vi "console_panel.vi"() -> ()   [LabVIEW 2012]
doc: "This VI is to serve as a simplified version of the utility_panel.vi, demonstrating primarily the ability to communicate with the connected device via the ASCII commandset.\n\nProduced By:\n\nChristopher Lemieux\nKod Integrations, LLC\n4835 Marianne Drive\nMount Airy, MD 21771\nhttp://www.kodintegrations.com\nemail: clemieux@kodintegrations.com\nphone: (240) 687-1288"
uses:
  support/controls/utility_actions.ctl
  main_functions/commands.ctl
  support/controls/errors_actions.ctl
panel:
  in  "help":bool
  out "response":string
  in  "terminate":bool
  in  "raw_cmd":string
  in  "write_cmd":bool
  out "error out":errorcluster
  in  "error in (no error)":errorcluster
  # "COMMAND:"
  # "RESPONSE:"
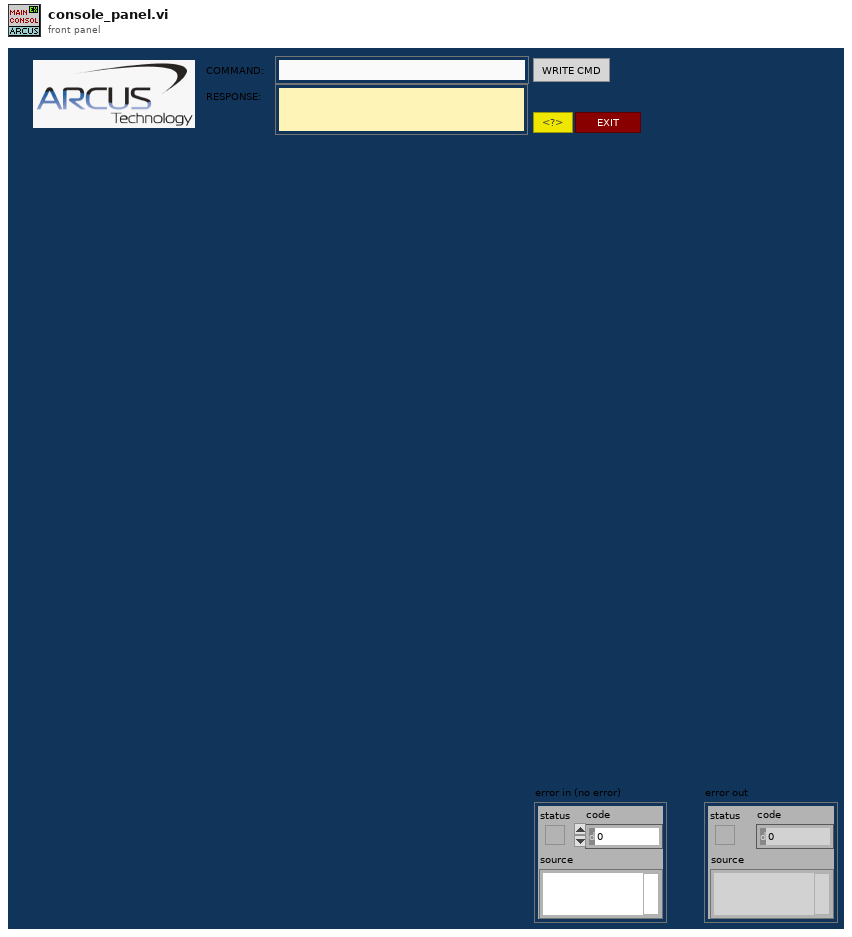
[diagram p1: front panel]
types:
  T1 = typedef "utility_actions.ctl" = enum16{"about", "clearError", "closeRef", "demo", "getAcceleration", "getActualCurrentVal", "getDeviceId", "getDeviceList", "getDigInputs", "getDigOutputs", "getDriverPowerStatus", "getFirmwareVer", "getHighSpeed", "getIdleCurrent", "getLowSpeed", "getMode", "getPolarity", "getPosition", "getProductId", "getRunCurrent", "getStatus", "homeMotorNeg", "homeMotorPos", "initialize", "jogConstNeg", "jogConstPos", "moveToPos", "openRef", "pause", "powerOFF", "powerON", "processEvents", "rawCmd", "setAcceleration", "setDeviceId", "setDigOutput", "setHighSpeed", "setLowSpeed", "setPolarity", "setPosition", "setRunCurrent", "setIdleCurrent", "setMode", "setTimeOuts", "stopImmediately", "stopSlowly", "storeToFlashMem", "updatePanelItems", "validateDemoPos", "validatePos", "waitUntilDone", "zeroPosition"}
  T2 = typedef "errors_actions.ctl" = enum16{"clearBuff", "closeRef", "noDeviceInfo", "noDevices", "openRef", "sendReceive", "setTimeouts", "unknown"}
  T3 = typedef "commands.ctl" = enum16{"clear error", "constant jog(-)", "constant jog(+)", "get acceleration", "get actual current", "get device id", "get digital input status", "get digial inputs status", "get dig output status", "get digital outputs status", "get firmware ver", "get high speed", "get idle current", "get low speed", "get micro step", "get motor status", "get move mode", "get polarity", "get position", "get product id", "get power status", "get run current", "get status", "home(-)", "home(+)", "move to position", "power down", "power up", "set acceleration", "set device id", "set digital output", "set digital outputs", "set high speed", "set idle current", "set low speed", "set move mode absolute", "set move mode increment", "set polarity", "set position", "set run current", "stop immediate", "stop slow", "store to memory"}
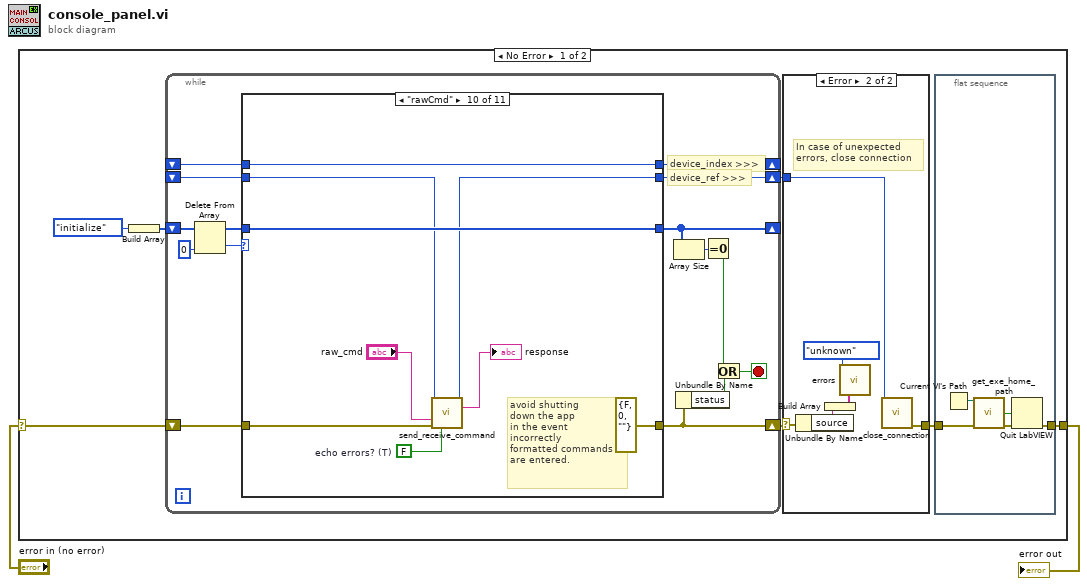
[diagram p0: block diagram]
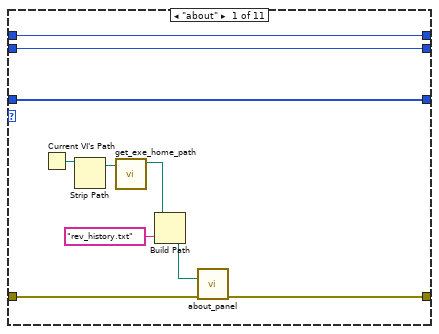
[diagram p3: hidden frame]
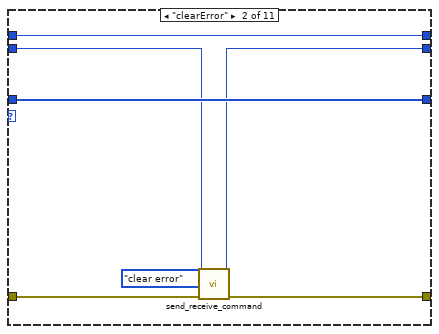
[diagram p4: hidden frame]
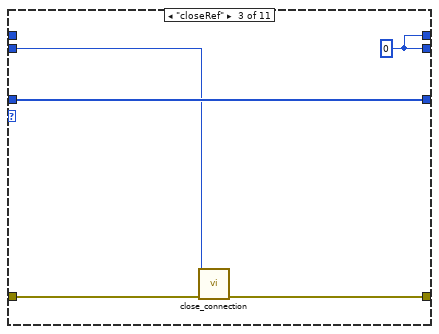
[diagram p5: hidden frame]
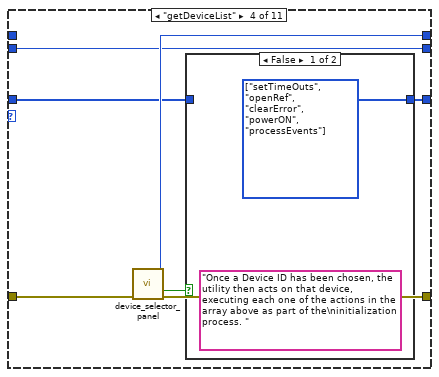
[diagram p6: hidden frame]
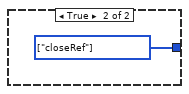
[diagram p7: hidden frame]
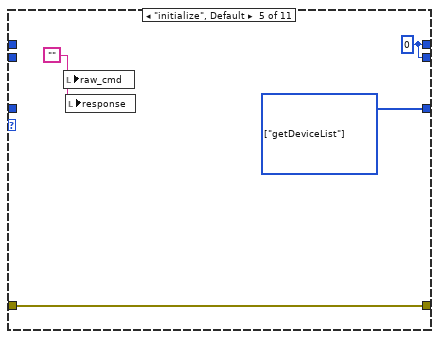
[diagram p8: hidden frame]
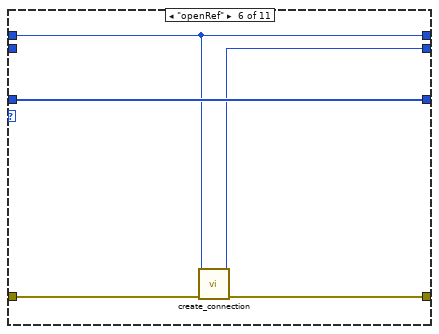
[diagram p9: hidden frame]
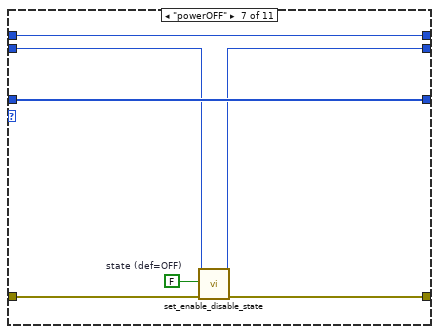
[diagram p10: hidden frame]
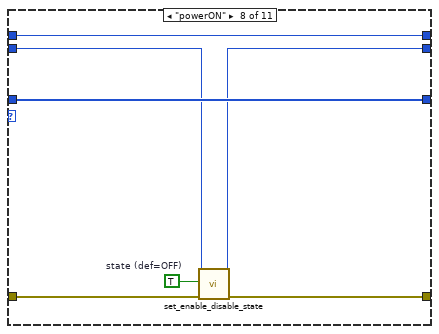
[diagram p11: hidden frame]
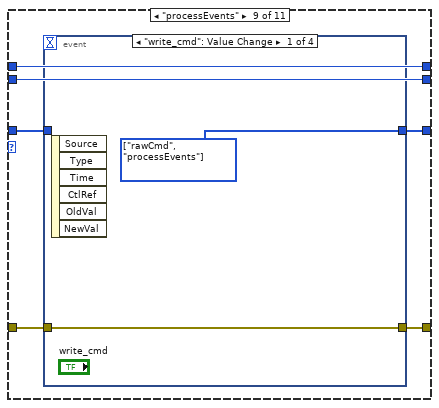
[diagram p12: hidden frame]
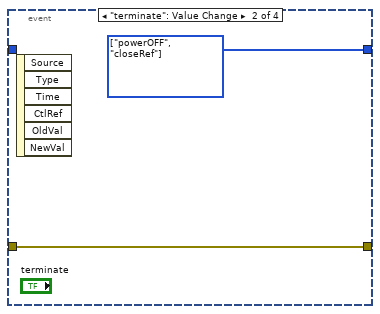
[diagram p13: hidden frame]
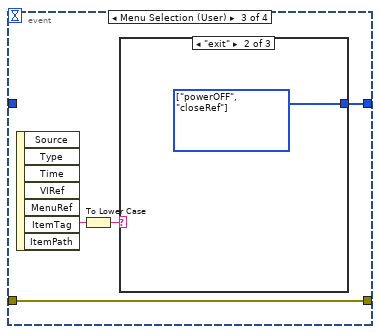
[diagram p14: hidden frame]
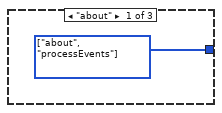
[diagram p15: hidden frame]
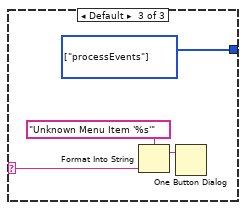
[diagram p16: hidden frame]
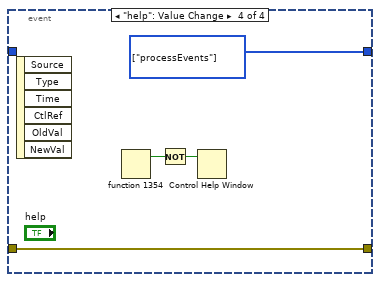
[diagram p17: hidden frame]
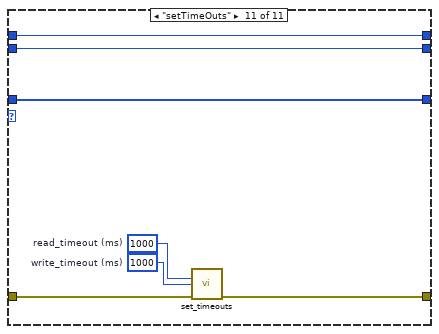
[diagram p18: hidden frame]
diagram:
  n1 = case shown="No Error" "error in (no error)" {
    selector: "error in (no error)" -> [w5 w129]
    tunnel: [w3 w129] -> w1
    frame No Error {
      n2 = Build Array(utility_actions."initialize" ("Enum")) -> (w8:T1[])
      n3 = while {
        shift-right: [w29] -> _
        shift-left: w8 -> [w34]
        shift-right: [w24] -> w7
        shift-left: w5 -> [w30]
        shift-right: [w23] -> w6
        shift-left: _ -> [w22]
        shift-right: [w21] -> _
        shift-left: _ -> [w20]
        stop <- w25 stop-if-true
        # "device_index >>>"
        # "device_ref >>>"
        n4 = Delete From Array(array=w34, index=0) -> (deleted portion=w32:T1, array with subset deleted=w31:T1[])  [unwired: 1 in]
        n5 = case shown="\"rawCmd\"" w32 {
          tunnel: w31 -> [w44 w51 w56 w58 _ w74 w81 w88 w91 w120 w122]
          tunnel: [w44 w51 w56 w57 w68 w74 w81 w88 w92 w120 w122] -> w29
          tunnel: w30 -> [w41 w49 w55 w63 w69 w73 w78 w86 w94 w121 w126]
          tunnel: [w40 w48 w54 w62 w69 w72 w77 w85 w93 errorcluster {"status"=FALSE, "code"=0, "source"=""} w125] -> w24
          tunnel: [w42 w46 w52 w60 w67 w71 w75 w82 w89 w115 w127] -> w23
          tunnel: w22 -> [w42 w47 w53 w60 _ _ w76 w83 w89 w116 w127]
          tunnel: [w43 w50 w52 w61 w67 w70 w80 w87 w90 w117 w128] -> w21
          tunnel: w20 -> [w43 w50 _ _ _ w70 w80 w87 w90 w117 w128]
          frame "about" {
            n6 = Current VI's Path() -> (path=w37:path)
            n7 = Strip Path(path=w37) -> (stripped path=w36:path)  [unwired: 1 out]
            n8 = call "get_exe_home_path.vi"("home_path"=w36) -> ("actual_home_path"=w35:path)  [unwired: 6 in, 1 out]
            n9 = Build Path(base path=w35, name or relative path="rev_history.txt") -> (appended path=w38:path)
            n10 = call "about_panel.vi"("rev_history_filepath"=w38, "error in (no error)"=w41) -> ("error out"=w40:errorcluster)  [unwired: 13 in]
          }
          frame "clearError" {
            n11 = call "send_receive_command.vi"("reference (in)"=w47, "command"=commands."clear error" ("commands"), "error in (no error)"=w49) -> ("reference (dup)"=w46:i32, "error out"=w48:errorcluster)  [unwired: 8 in, 3 out]
          }
          frame "closeRef" {
            w52 = 0 ("reference (out)")
            n12 = call "close_connection.vi"("reference"=w53, "error in (no error)"=w55) -> ("error out"=w54:errorcluster)  [unwired: 13 in]
          }
          frame "getDeviceList" {
            n13 = call "device_selector_panel.vi"("error in (no error)"=w63) -> ("index"=w61:i32, "cancel?"=w59:bool, "error out"=w62:errorcluster)  [unwired: 10 in, 2 out]
            n14 = case shown="False" w59 {
              tunnel: w58 -> [_ _]
              tunnel: [w64 w65] -> w57
              frame False {
                w64 = T1[] [enum."setTimeOuts", enum."openRef", enum."clearError", enum."powerON", enum."processEvents"] items=["about", "clearError", "closeRef", "demo", "getAcceleration", "getActualCurrentVal", "getDeviceId", "getDeviceList", "getDigInputs", "getDigOutputs", "getDriverPowerStatus", "getFirmwareVer", "getHighSpeed", "getIdleCurrent", "getLowSpeed", "getMode", "getPolarity", "getPosition", "getProductId", "getRunCurrent", "getStatus", "homeMotorNeg", "homeMotorPos", "initialize", "jogConstNeg", "jogConstPos", "moveToPos", "openRef", "pause", "powerOFF", "powerON", "processEvents", "rawCmd", "setAcceleration", "setDeviceId", "setDigOutput", "setHighSpeed", "setLowSpeed", "setPolarity", "setPosition", "setRunCurrent", "setIdleCurrent", "setMode", "setTimeOuts", "stopImmediately", "stopSlowly", "storeToFlashMem", "updatePanelItems", "validateDemoPos", "validatePos", "waitUntilDone", "zeroPosition"] ("actions")
                (unwired) "Once a Device ID has been chosen, the utility then acts on that device, executing each one of the actions in the array above as part of the\ninitialization process. "
              }
              frame True {
                w65 = T1[] [enum."closeRef"] items=["about", "clearError", "closeRef", "demo", "getAcceleration", "getActualCurrentVal", "getDeviceId", "getDeviceList", "getDigInputs", "getDigOutputs", "getDriverPowerStatus", "getFirmwareVer", "getHighSpeed", "getIdleCurrent", "getLowSpeed", "getMode", "getPolarity", "getPosition", "getProductId", "getRunCurrent", "getStatus", "homeMotorNeg", "homeMotorPos", "initialize", "jogConstNeg", "jogConstPos", "moveToPos", "openRef", "pause", "powerOFF", "powerON", "processEvents", "rawCmd", "setAcceleration", "setDeviceId", "setDigOutput", "setHighSpeed", "setLowSpeed", "setPolarity", "setPosition", "setRunCurrent", "setIdleCurrent", "setMode", "setTimeOuts", "stopImmediately", "stopSlowly", "storeToFlashMem", "updatePanelItems", "validateDemoPos", "validatePos", "waitUntilDone", "zeroPosition"] ("actions")
              }
            }
          }
          frame "initialize", Default {
            w68 = T1[] [enum."getDeviceList"] items=["about", "clearError", "closeRef", "demo", "getAcceleration", "getActualCurrentVal", "getDeviceId", "getDeviceList", "getDigInputs", "getDigOutputs", "getDriverPowerStatus", "getFirmwareVer", "getHighSpeed", "getIdleCurrent", "getLowSpeed", "getMode", "getPolarity", "getPosition", "getProductId", "getRunCurrent", "getStatus", "homeMotorNeg", "homeMotorPos", "initialize", "jogConstNeg", "jogConstPos", "moveToPos", "openRef", "pause", "powerOFF", "powerON", "processEvents", "rawCmd", "setAcceleration", "setDeviceId", "setDigOutput", "setHighSpeed", "setLowSpeed", "setPolarity", "setPosition", "setRunCurrent", "setIdleCurrent", "setMode", "setTimeOuts", "stopImmediately", "stopSlowly", "storeToFlashMem", "updatePanelItems", "validateDemoPos", "validatePos", "waitUntilDone", "zeroPosition"] ("actions")
            w67 = 0 ("index")
            w66 = ""
            n15 = local write "raw_cmd"(w66) -> ()
            n16 = local write "response"(w66) -> ()
          }
          frame "openRef" {
            n17 = call "create_connection.vi"("device_index (def=0)"=w70, "error in (no error)"=w73) -> ("reference"=w71:i32, "error out"=w72:errorcluster)  [unwired: 12 in]
          }
          frame "powerOFF" {
            w79 = FALSE  # state (def=OFF)
            n18 = call "set_enable_disable_state.vi"("reference (in)"=w76, "state (def=OFF)"=w79, "error in (no error)"=w78) -> ("reference (dup)"=w75:i32, "error out"=w77:errorcluster)  [unwired: 14 in, 1 out]
          }
          frame "powerON" {
            w84 = TRUE  # state (def=OFF)
            n19 = call "set_enable_disable_state.vi"("reference (in)"=w83, "state (def=OFF)"=w84, "error in (no error)"=w86) -> ("reference (dup)"=w82:i32, "error out"=w85:errorcluster)  [unwired: 14 in, 1 out]
          }
          frame "processEvents" {
            n20 = event shown="[0] \"write_cmd\": Value Change" {
              selector: _ -> [_ _ _ _]
              dyn-events: _ -> [_ _ _ _]
              timeout: _ -> [_ _ _ _]
              tunnel: [w96 w98 w99 w112] -> w93
              tunnel: w94 -> [w96 w98 w99 w112]
              tunnel: [w95 w97 w100 w111] -> w92
              tunnel: w91 -> [_ _ _ _]
              event "write_cmd": Value Change {
                w95 = T1[] [enum."rawCmd", enum."processEvents"] items=["about", "clearError", "closeRef", "demo", "getAcceleration", "getActualCurrentVal", "getDeviceId", "getDeviceList", "getDigInputs", "getDigOutputs", "getDriverPowerStatus", "getFirmwareVer", "getHighSpeed", "getIdleCurrent", "getLowSpeed", "getMode", "getPolarity", "getPosition", "getProductId", "getRunCurrent", "getStatus", "homeMotorNeg", "homeMotorPos", "initialize", "jogConstNeg", "jogConstPos", "moveToPos", "openRef", "pause", "powerOFF", "powerON", "processEvents", "rawCmd", "setAcceleration", "setDeviceId", "setDigOutput", "setHighSpeed", "setLowSpeed", "setPolarity", "setPosition", "setRunCurrent", "setIdleCurrent", "setMode", "setTimeOuts", "stopImmediately", "stopSlowly", "storeToFlashMem", "updatePanelItems", "validateDemoPos", "validatePos", "waitUntilDone", "zeroPosition"] ("actions")
                n21 = event-data() -> ()  [unwired: 1 in, 6 out]
              }
              event "terminate": Value Change {
                w97 = T1[] [enum."powerOFF", enum."closeRef"] items=["about", "clearError", "closeRef", "demo", "getAcceleration", "getActualCurrentVal", "getDeviceId", "getDeviceList", "getDigInputs", "getDigOutputs", "getDriverPowerStatus", "getFirmwareVer", "getHighSpeed", "getIdleCurrent", "getLowSpeed", "getMode", "getPolarity", "getPosition", "getProductId", "getRunCurrent", "getStatus", "homeMotorNeg", "homeMotorPos", "initialize", "jogConstNeg", "jogConstPos", "moveToPos", "openRef", "pause", "powerOFF", "powerON", "processEvents", "rawCmd", "setAcceleration", "setDeviceId", "setDigOutput", "setHighSpeed", "setLowSpeed", "setPolarity", "setPosition", "setRunCurrent", "setIdleCurrent", "setMode", "setTimeOuts", "stopImmediately", "stopSlowly", "storeToFlashMem", "updatePanelItems", "validateDemoPos", "validatePos", "waitUntilDone", "zeroPosition"] ("actions")
                n22 = event-data() -> ()  [unwired: 1 in, 6 out]
              }
              event Menu Selection (User) {
                n23 = event-data() -> ("ItemTag"=w102:string)  [unwired: 1 in, 6 out]
                n24 = To Lower Case(string=w102) -> (all lower case string=w101:string)
                n25 = case shown="\"exit\"" w101 {
                  selector: w101 -> [_ _ w105]
                  tunnel: [w103 w104 w108] -> w100
                  frame "about" {
                    w103 = T1[] [enum."about", enum."processEvents"] items=["about", "clearError", "closeRef", "demo", "getAcceleration", "getActualCurrentVal", "getDeviceId", "getDeviceList", "getDigInputs", "getDigOutputs", "getDriverPowerStatus", "getFirmwareVer", "getHighSpeed", "getIdleCurrent", "getLowSpeed", "getMode", "getPolarity", "getPosition", "getProductId", "getRunCurrent", "getStatus", "homeMotorNeg", "homeMotorPos", "initialize", "jogConstNeg", "jogConstPos", "moveToPos", "openRef", "pause", "powerOFF", "powerON", "processEvents", "rawCmd", "setAcceleration", "setDeviceId", "setDigOutput", "setHighSpeed", "setLowSpeed", "setPolarity", "setPosition", "setRunCurrent", "setIdleCurrent", "setMode", "setTimeOuts", "stopImmediately", "stopSlowly", "storeToFlashMem", "updatePanelItems", "validateDemoPos", "validatePos", "waitUntilDone", "zeroPosition"] ("actions")
                  }
                  frame "exit" {
                    w104 = T1[] [enum."powerOFF", enum."closeRef"] items=["about", "clearError", "closeRef", "demo", "getAcceleration", "getActualCurrentVal", "getDeviceId", "getDeviceList", "getDigInputs", "getDigOutputs", "getDriverPowerStatus", "getFirmwareVer", "getHighSpeed", "getIdleCurrent", "getLowSpeed", "getMode", "getPolarity", "getPosition", "getProductId", "getRunCurrent", "getStatus", "homeMotorNeg", "homeMotorPos", "initialize", "jogConstNeg", "jogConstPos", "moveToPos", "openRef", "pause", "powerOFF", "powerON", "processEvents", "rawCmd", "setAcceleration", "setDeviceId", "setDigOutput", "setHighSpeed", "setLowSpeed", "setPolarity", "setPosition", "setRunCurrent", "setIdleCurrent", "setMode", "setTimeOuts", "stopImmediately", "stopSlowly", "storeToFlashMem", "updatePanelItems", "validateDemoPos", "validatePos", "waitUntilDone", "zeroPosition"] ("actions")
                  }
                  frame Default {
                    w108 = T1[] [enum."processEvents"] items=["about", "clearError", "closeRef", "demo", "getAcceleration", "getActualCurrentVal", "getDeviceId", "getDeviceList", "getDigInputs", "getDigOutputs", "getDriverPowerStatus", "getFirmwareVer", "getHighSpeed", "getIdleCurrent", "getLowSpeed", "getMode", "getPolarity", "getPosition", "getProductId", "getRunCurrent", "getStatus", "homeMotorNeg", "homeMotorPos", "initialize", "jogConstNeg", "jogConstPos", "moveToPos", "openRef", "pause", "powerOFF", "powerON", "processEvents", "rawCmd", "setAcceleration", "setDeviceId", "setDigOutput", "setHighSpeed", "setLowSpeed", "setPolarity", "setPosition", "setRunCurrent", "setIdleCurrent", "setMode", "setTimeOuts", "stopImmediately", "stopSlowly", "storeToFlashMem", "updatePanelItems", "validateDemoPos", "validatePos", "waitUntilDone", "zeroPosition"] ("actions")
                    n26 = Format Into String(format string="Unknown Menu Item '%s'" ("message"), w105) -> (resulting string=w106:string)  [unwired: 2 in, 1 out]
                    n27 = One Button Dialog(message=w106) -> ()  [unwired: 1 in, 1 out]
                  }
                }
              }
              event "help": Value Change {
                w111 = T1[] [enum."processEvents"] items=["about", "clearError", "closeRef", "demo", "getAcceleration", "getActualCurrentVal", "getDeviceId", "getDeviceList", "getDigInputs", "getDigOutputs", "getDriverPowerStatus", "getFirmwareVer", "getHighSpeed", "getIdleCurrent", "getLowSpeed", "getMode", "getPolarity", "getPosition", "getProductId", "getRunCurrent", "getStatus", "homeMotorNeg", "homeMotorPos", "initialize", "jogConstNeg", "jogConstPos", "moveToPos", "openRef", "pause", "powerOFF", "powerON", "processEvents", "rawCmd", "setAcceleration", "setDeviceId", "setDigOutput", "setHighSpeed", "setLowSpeed", "setPolarity", "setPosition", "setRunCurrent", "setIdleCurrent", "setMode", "setTimeOuts", "stopImmediately", "stopSlowly", "storeToFlashMem", "updatePanelItems", "validateDemoPos", "validatePos", "waitUntilDone", "zeroPosition"] ("actions")
                n28 = event-data() -> ()  [unwired: 1 in, 6 out]
                n29 = fn#1354() -> (1:w110:bool)  [unwired: 1 out]
                n30 = Not(x=w110) -> (.not. x?=w109:bool)
                n31 = Control Help Window(1:w109) -> ()  [unwired: 1 in]
              }
            }
          }
          frame "rawCmd" {
            w113 = FALSE  # echo errors? (T)
            # "avoid shutting\ndown the app\nin the event\nincorrectly \nformatted commands\nare entered."
            n32 = call "send_receive_command.vi"("reference (in)"=w116, "command (raw)"="raw_cmd", "error in (no error)"=w121, "echo errors? (T)"=w113) -> ("reference (dup)"=w115:i32, "read_string"=→"response":string)  [unwired: 7 in, 3 out]
          }
          frame "setTimeOuts" {
            w123 = 1000  # write_timeout (ms)
            w124 = 1000  # read_timeout (ms)
            n33 = call "set_timeouts.vi"("read_timeout (ms); def=1000"=w124, "write_timeout (ms); def=1000"=w123, "error in (no error)"=w126) -> ("error out"=w125:errorcluster)  [unwired: 12 in]
          }
        }
        n34 = Array Size(array=w29) -> (size(s)=w28:i32)
        n35 = Unbundle By Name(w24) -> ("status"=w26:bool)
        n36 = Equal To 0?(x=w28) -> (x = 0?=w27:bool)
        n37 = Or(x=w27, y=w26) -> (x .or. y?=w25:bool)
      }
      n38 = case shown="Error" w7 {
        selector: w7 -> [w13 w16]
        tunnel: w6 -> [_ w19]
        tunnel: [w13 w18] -> w4
        frame No Error {
        }
        frame Error {
          # "In case of unexpected\nerrors, close connection"
          n39 = Unbundle By Name(w16) -> ("source"=w15:string)
          n40 = Build Array(w15) -> (w14:string[])
          n41 = call "errors.vi"("errors"=errors_actions."unknown", "supp_text"=w14) -> ()  [unwired: 13 in, 1 out]
          n42 = call "close_connection.vi"("reference"=w19) -> ("error out"=w18:errorcluster)  [unwired: 14 in]
        }
      }
      n43 = flat-sequence {
        tunnel: w4 -> [w10]
        tunnel: [w10] -> w3
        frame #0 {
          n44 = Current VI's Path() -> (path=w12:path)
          n45 = call "get_exe_home_path.vi"("home_path"=w12) -> ("running in an executable?"=w11:bool)  [unwired: 6 in, 1 out]
          n46 = Quit LabVIEW(quit? (T)=w11) -> ()
        }
      }
    }
    frame Error {
    }
  }
  "error out" <- w1
